vi "RS_SMBV100A_PARS_SAT_TIME_AND_NUMBER.vi"(0 "Parsing Satelite":T1) -> (14 "OUT GNSS NUMBERACTIVESAT":dbl, 15 "GNSS 2D SAT":dbl[][](array[numeric]), 16 "OUT GPS NUMBERACTIVESAT":dbl, 17 "GPS 2D SAT":dbl[][](array[numeric]), 18 "OUT GLONASS NUMBERACTIVESAT":dbl, 19 "GLONASS 2D SAT":dbl[][](array[numeric]))   [LabVIEW 2018]
uses:
  RS_SMBV100A_Parsing Satelite.ctl
panel:
  # "Входные данные по спутникам"
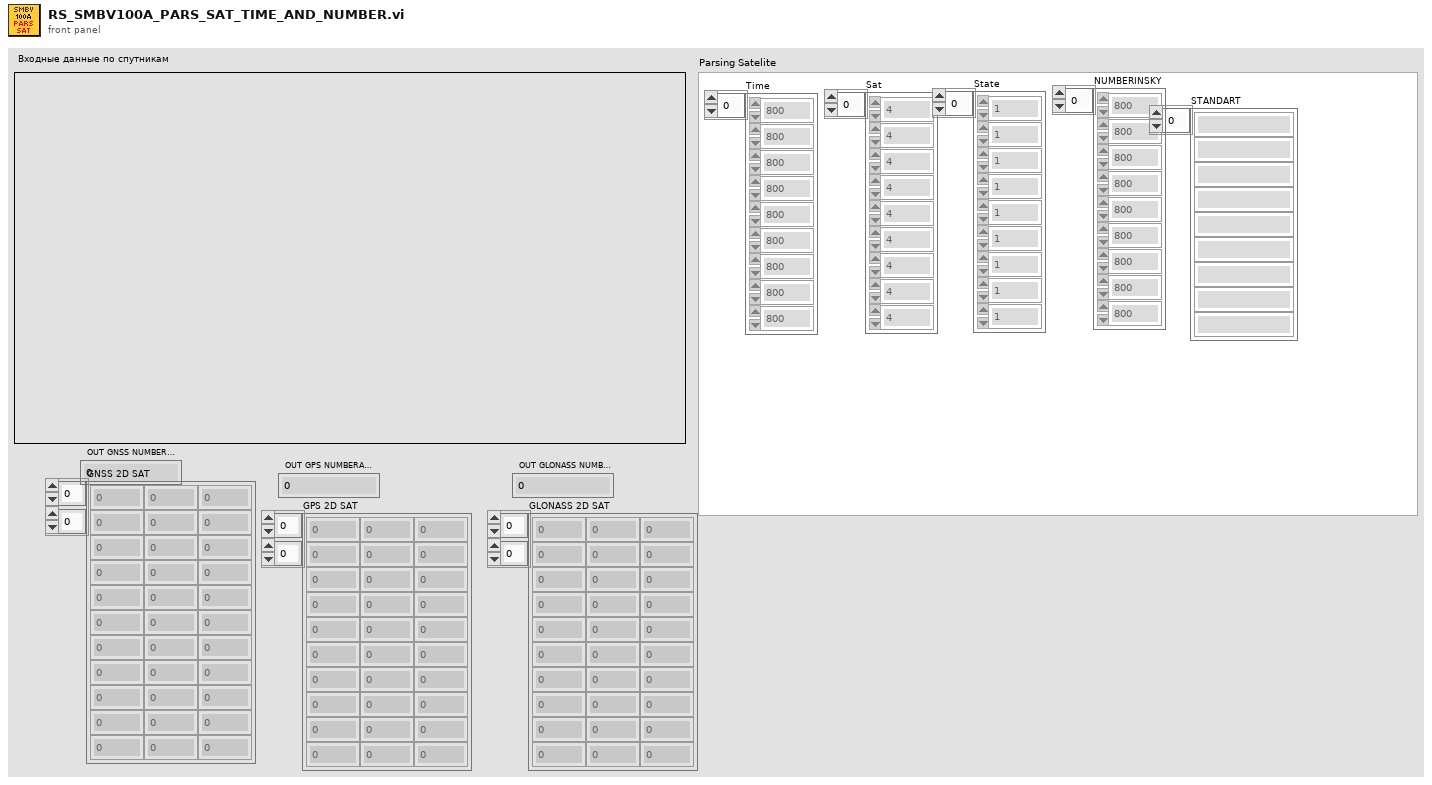
[diagram p1: front panel]
types:
  T1 = typedef "RS_SMBV100A_Parsing Satelite.ctl" = cluster{"Time":dbl[], "Sat":dbl[], "State":dbl[], "NUMBERINSKY":dbl[], "STANDART":string[]}
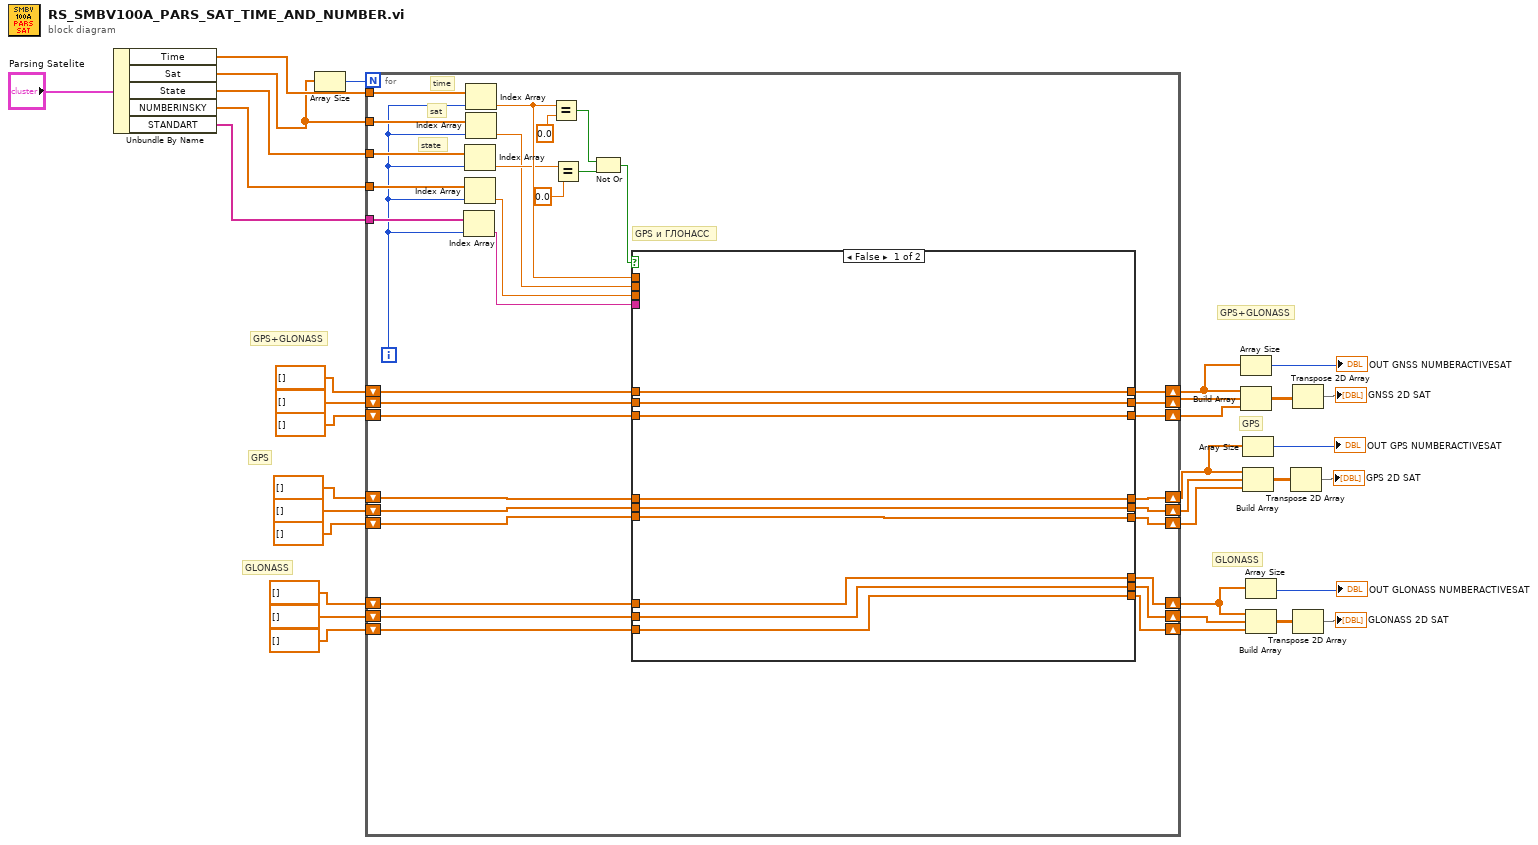
[diagram p0: block diagram]
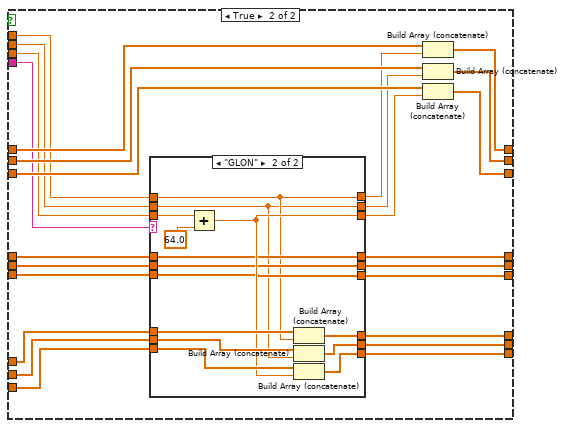
[diagram p2: hidden frame]
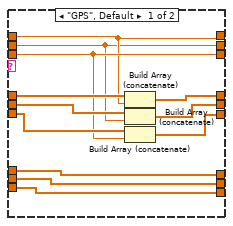
[diagram p3: hidden frame]
diagram:
  # "GLONASS"
  # "GPS"
  # "GPS+GLONASS"
  # "GLONASS"
  # "GPS"
  # "GPS+GLONASS"
  n1 = Unbundle By Name("Parsing Satelite") -> ("Time"=w5:dbl[], "Sat"=w4:dbl[], "State"=w3:dbl[], "NUMBERINSKY"=w2:dbl[], "STANDART"=w1:string[])
  n2 = Array Size(array=w4) -> (size(s)=w34:i32)
  n3 = for {
    N: w34 -> [_]
    tunnel: w5 -> [w68]
    tunnel: w4 -> [w67]
    tunnel: w3 -> [w66]
    shift-right: [w62] -> w22
    shift-left: dbl[] [] ("Array") -> [w61]
    shift-right: [w57] -> w24
    shift-left: dbl[] [] ("Array") -> [w56]
    tunnel: w2 -> [w55]
    tunnel: w1 -> [w54]
    shift-right: [w50] -> w23
    shift-left: dbl[] [] ("Array") -> [w49]
    shift-right: [w42] -> w16
    shift-left: dbl[] [] ("Array") -> [w48]
    shift-right: [w41] -> w21
    shift-left: dbl[] [] ("Array") -> [w47]
    shift-right: [w40] -> w20
    shift-left: dbl[] [] ("Array") -> [w46]
    shift-right: [w39] -> w18
    shift-left: dbl[] [] ("Array") -> [w45]
    shift-right: [w38] -> w19
    shift-left: dbl[] [] ("Array") -> [w44]
    shift-right: [w37] -> w17
    shift-left: dbl[] [] ("Array") -> [w43]
    i -> [w53]
    # "GPS и ГЛОНАСС"
    # "state"
    # "sat"
    # "time"
    n4 = Index Array(array=w54, index=w53) -> (element=w51:string)
    n5 = Index Array(array=w66, index=w53) -> (element=w59:dbl)
    n6 = Index Array(array=w55, index=w53) -> (element=w52:dbl)
    n7 = Index Array(array=w68, index=w53) -> (element=w60:dbl)
    n8 = Index Array(array=w67, index=w53) -> (element=w58:dbl)
    n9 = Equal?(x=w60, y=0.0) -> (x = y?=w64:bool)
    n10 = Equal?(x=w59, y=0.0) -> (x = y?=w63:bool)
    n11 = Not Or(1:w63, 2:w64) -> (0:w35:bool)
    n12 = case shown="False" w35 {
      tunnel: [w77 w102] -> w62
      tunnel: w61 -> [w77 w101]
      tunnel: w60 -> [_ w79]
      tunnel: w58 -> [_ w86]
      tunnel: [w76 w100] -> w57
      tunnel: w56 -> [w76 w99]
      tunnel: w52 -> [_ w95]
      tunnel: w51 -> [_ w96]
      tunnel: [w75 w98] -> w50
      tunnel: w49 -> [w75 w97]
      tunnel: w48 -> [w74 w93]
      tunnel: w47 -> [w73 w92]
      tunnel: w46 -> [w72 w91]
      tunnel: w45 -> [w71 w90]
      tunnel: w44 -> [w70 w89]
      tunnel: w43 -> [w69 w88]
      tunnel: [w74 w87] -> w42
      tunnel: [w73 w85] -> w41
      tunnel: [w72 w84] -> w40
      tunnel: [w71 w83] -> w39
      tunnel: [w70 w82] -> w38
      tunnel: [w69 w81] -> w37
      frame False {
      }
      frame True {
        n13 = case shown="\"GLON\"" w96 {
          tunnel: w95 -> [w110 w125]
          tunnel: [w110 w123] -> w94
          tunnel: w93 -> [w112 w122]
          tunnel: w92 -> [w114 w121]
          tunnel: w91 -> [w113 w120]
          tunnel: w90 -> [w107 w128]
          tunnel: w89 -> [w106 w127]
          tunnel: w88 -> [w105 w126]
          tunnel: w79 -> [w104 w116]
          tunnel: [w111 w122] -> w87
          tunnel: w86 -> [w103 w115]
          tunnel: [w109 w121] -> w85
          tunnel: [w108 w120] -> w84
          tunnel: [w107 w119] -> w83
          tunnel: [w106 w118] -> w82
          tunnel: [w105 w117] -> w81
          tunnel: [w104 w116] -> w78
          tunnel: [w103 w115] -> w80
          frame "GPS", Default {
            n14 = Build Array (concatenate)(w112, w104) -> (w111:dbl[])
            n15 = Build Array (concatenate)(w114, w103) -> (w109:dbl[])
            n16 = Build Array (concatenate)(w113, w110) -> (w108:dbl[])
          }
          frame "GLON" {
            n17 = Add(x=64.0 ("y"), y=w125) -> (x+y=w123:dbl)
            n18 = Build Array (concatenate)(w128, w116) -> (w119:dbl[])
            n19 = Build Array (concatenate)(w127, w115) -> (w118:dbl[])
            n20 = Build Array (concatenate)(w126, w123) -> (w117:dbl[])
          }
        }
        n21 = Build Array (concatenate)(w101, w78) -> (w102:dbl[])
        n22 = Build Array (concatenate)(w99, w80) -> (w100:dbl[])
        n23 = Build Array (concatenate)(w97, w94) -> (w98:dbl[])
      }
    }
  }
  n24 = Array Size(array=w22) -> (size(s)=→"OUT GNSS NUMBERACTIVESAT":i32)
  n25 = Build Array(w22, w24, w23) -> (w15:dbl[][])
  n26 = Array Size(array=w16) -> (size(s)=→"OUT GPS NUMBERACTIVESAT":i32)
  n27 = Build Array(w16, w21, w20) -> (w10:dbl[][])
  n28 = Array Size(array=w18) -> (size(s)=→"OUT GLONASS NUMBERACTIVESAT":i32)
  n29 = Build Array(w18, w19, w17) -> (w11:dbl[][])
  n30 = Transpose 2D Array(2D array=w10) -> (transposed array=→"GPS 2D SAT":dbl[][])
  n31 = Transpose 2D Array(2D array=w15) -> (transposed array=→"GNSS 2D SAT":dbl[][])
  n32 = Transpose 2D Array(2D array=w11) -> (transposed array=→"GLONASS 2D SAT":dbl[][])
